vi "Get Instrument Addon Name.vi"(8 "Error In":errorcluster, 11 "Instrument Addon Refnum In":T1 format="%.0x") -> (0 "Error Out":errorcluster, 2 "Name":string, 3 "Instrument Addon Refnum Out":T1=18446744073709551615 format="%.0x")   [LabVIEW 2018, in "Instrument Addon Scripting API.lvlib"]
doc: "Returns the name of an Instrument Addon Custom Device\n\nInput:\nInstrument Addon Refnum In: the refference number (NodeID) of a Custom Device\n\nOutput: \nInstrument Addon Refnum Out: the Instrument Addon Custom Device refference number provided as input\nName: represents the name of the Custom Device"
uses:
  Instrument Addon Scripting API.lvlib
  <vilib>/NI Veristand/Custom Device API/Custom Device Item Ref.ctl
  <vilib>/Utility/error.llb/Error Cluster From Error Code.vi
  <vilib>/ErrorRing/Error Ring.xnode
  <vilib>/NI/NI VeriStand Advanced SysDef API/SysDef API/Advanced System Definition.lvlib
  <vilib>/NI Veristand/Custom Device API/Custom Device API.lvlib
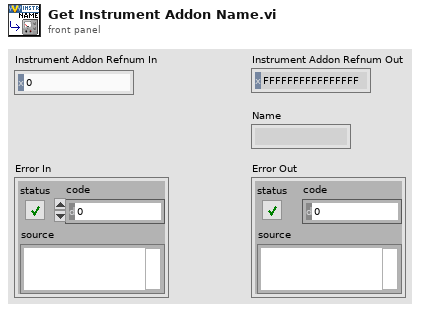
[diagram p1: front panel]
types:
  T1 = typedef "Custom Device API.lvlib/Custom Device Item Ref.ctl" = u64
  T2 = typedef "Advanced System Definition.lvlib/TreeItem.Info.ctl" = cluster{"Name":string, "Description":string, "GUID":string, "Is Channel":bool, "Channel":T3, "Is Waveform":bool, "Waveform":T5}
  T3 = typedef "Custom Device API.lvlib/Custom Device Channel.ctl" = cluster{"Type":T4, "Units":string, "Default Value":dbl, "Faultable":bool, "Scalable":bool}
  T4 = typedef "Custom Device API.lvlib/Custom Device Channel Type.ctl" = enum16{"Input", "Output"}
  T5 = typedef "Custom Device API.lvlib/Custom Device Waveform.ctl" = cluster{"Data Type":T6, "Units":string}
  T6 = typedef "Custom Device API.lvlib/Custom Device Waveform DataType.ctl" = enum16{"Double", "Complex Double"}
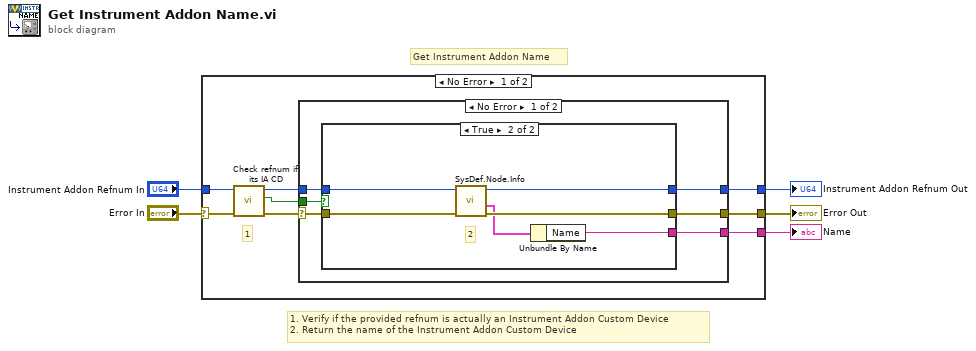
[diagram p0: block diagram]
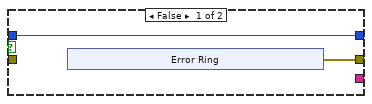
[diagram p2: hidden frame]
diagram:
  # "1. Verify if the provided refnum is actually an Instrument Addon Custom Device\n2. Return the name of the Instrument Addon Custom Device"
  # "Get Instrument Addon Name"
  n1 = case shown="No Error" "Error In" {
    selector: "Error In" -> [w12 w36]
    tunnel: "Instrument Addon Refnum In" -> [w13 w35]
    tunnel: [w9 w36] -> w4
    tunnel: [w8 w35] -> w2
    tunnel: [w7 _] -> w1
    frame No Error {
      # "1"
      n2 = call "Check refnum if its IA CD.vi"("Error In"=w12, "Refnum In"=w13) -> ("Error Out"=w6:errorcluster, "Is Instrument Addon?"=w11:bool, "Refnum Out"=w10:u64)  [unwired: 7 in]
      n3 = case shown="No Error" w6 {
        selector: w6 -> [w14 w34]
        tunnel: w11 -> [w19 _]
        tunnel: w10 -> [w18 w33]
        tunnel: [w17 w34] -> w9
        tunnel: [w16 w33] -> w8
        tunnel: [w15 _] -> w7
        frame No Error {
          n4 = case shown="True" w19 {
            tunnel: w18 -> [w20 w32]
            tunnel: [w21 w31] -> w17
            tunnel: [w20 w30] -> w16
            tunnel: [_ w28] -> w15
            tunnel: w14 -> [_ w27]
            frame False {
              n5 = xnode "Error Ring"() -> ("error out"=w21:errorcluster)
            }
            frame True {
              # "2"
              n6 = call <vilib>:"SysDef.Node.Info.vi"("error in (no error)"=w27, "nodeID"=w32) -> ("error out"=w31:errorcluster, "Item Info"=w29:T2, "nodeID out"=w30:u64)  [unwired: 6 in, 1 out]
              n7 = Unbundle By Name(w29) -> ("Name"=w28:string)
            }
          }
        }
        frame Error {
        }
      }
    }
    frame Error {
    }
  }
  "Error Out" <- w4
  "Instrument Addon Refnum Out" <- w2
  "Name" <- w1
